vi "Read Database Settings.vi"(8 "error in (no error)":errorcluster, 11 "AcPwrSimBase in":refnum<class "AcPwrSimBase.lvclass">) -> (0 "error out":errorcluster, 2 "Database Settings":T1, 3 "AcPwrSimBase out":refnum<class "AcPwrSimBase.lvclass">)   [LabVIEW 2018, in "AcPwrPlugins.lvlib" / "AcPwrSimBase.lvclass"]
uses:
  AcPwrSimBase.lvclass
  AcPwrShared/Database Settings.ctl
  AcPwrShared/AcPwrShared.lvlib
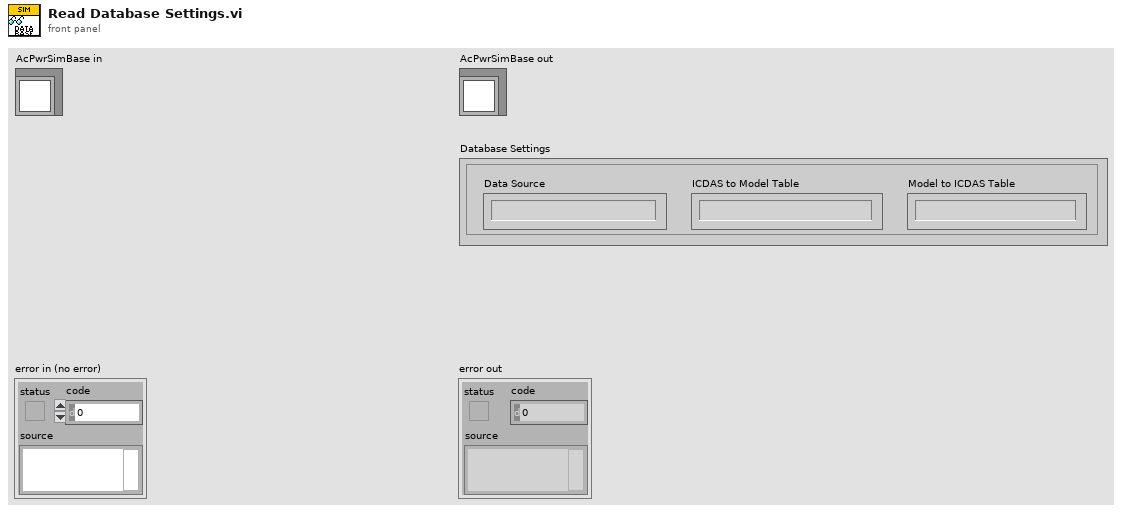
[diagram p1: front panel]
types:
  T1 = typedef "AcPwrShared.lvlib/Database Settings.ctl" = cluster{"Data Source":string, "ICDAS to Model Table":string, "Model to ICDAS Table":string}
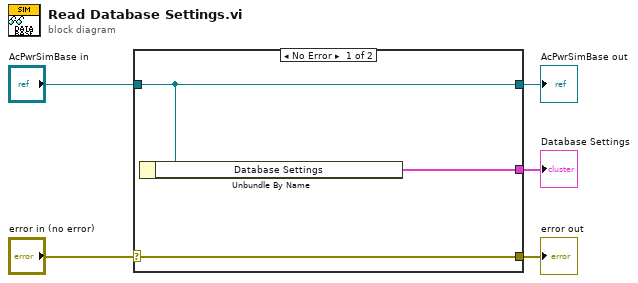
[diagram p0: block diagram]
diagram:
  n1 = case shown="No Error" "error in (no error)" {
    selector: "error in (no error)" -> [w8 w9]
    tunnel: [w8 w9] -> w4
    tunnel: [w7 w10] -> w2
    tunnel: "AcPwrSimBase in" -> [w7 w10]
    tunnel: [w6 _] -> w1
    frame No Error {
      n2 = Unbundle By Name(w7) -> ("Database Settings"=w6:T1)
    }
    frame Error {
    }
  }
  "error out" <- w4
  "AcPwrSimBase out" <- w2
  "Database Settings" <- w1
